vi "Set UI.vi"(6 "Lock":bool, 8 "error in (no error)":errorcluster, 10 "Available Tests":T6, 11 "Cluster":T1={"Queue Array"=[], "Queue Element"={"state"="", "data"=variant}, "System Event"=refnum, "System Event RefNum"=refnum, "Queue List"=[], "LPCA COM"="", "Rotating"=FALSE, "PrecorAI"="", "T_0 Index"=0, "Bar Graph X"=[], "Channels"=[], "Active Indicies"=[], "Active Channels"=[], "Sample Frequency"=0.0, "Ibrake Sweep"=[], "RPM Sweep"=[], "Load Sweep"=[], "Step Height Sweep"=[], "Range Sweep"=[], "A Counter"=0, "B Counter"=0, "C Counter"=0, "#A"=0, "#B"=0, "#C"=0, "Current RPM"=0.0, "Current Ibrake"=0, "Current Range"=0, "Current Step Height"=0, "Load Bank"=enum."OFF", "Cfg Cntrls"=[], "T_Monitor Indices"=[], "Thermal Limit"=0, "Thermal Resume"=0, "Timer Reset"=FALSE, "Stop Time"=0.0, "Autotest"=FALSE, "Pulsed RPM Capture"=FALSE, "Get Sample"=FALSE, "Last State"="", "Reset Timeout"=FALSE, "Ctrl Refs"={"Test Details"=refnum, "Save Config"=refnum, "Load Config"=refnum, "Path"=refnum, "Snapshot"=refnum, "SS#"=refnum, "Ibrake"=refnum, "RPM Target"=refnum, "Spin"=refnum, "Load Bank"=refnum, "Start Test"=refnum, "Pause Test"=refnum, "Load Sweep"=refnum, "RPM Sweep"=refnum, "Ibrake Sweep"=refnum, "Filters"=refnum, "Sample Frequency"=refnum, "Data Setup"=refnum, "Pause"=refnum, "Stop Time"=refnum, "S Period"=refnum, "Range"=refnum, "Step Height"=refnum, "Step Height Sweep"=refnum, "Range Sweep"=refnum, "Available Tests"=refnum, "RPM Graph"=refnum, "RPM Knob"=refnum, "FanMode"=refnum, "Fan Mode LED Array"=refnum, "Thermal Equilibrium"=refnum, "Data Display"=refnum, "LPCA Error"=refnum, "LPCA Ramp"=refnum, "LPCA Range"=refnum, "LPCA Resistance"=refnum, "Analyze Read"=refnum, "Console Select"=refnum, "Sub Panel"=refnum}, "Pulse Waveform"={"t0"=timestamp(0 s since 1904-01-01), "dt"=1.0, "Y"=[]}, "Snapshot"={"Test Details"="test", "Version"="test", "Date"=timestamp(3493915594.3018084 s since 1904-01-01), "Selected Test"="man", "Snapshot Number"=0, "Time"=timestamp(3493915602.7292905 s since 1904-01-01), "Ibrake Setpoint"="1", "RPM Setpoint"="20", "Range Setpoint"="", "Step Height Setpoint"="", "Load Bank Setpoint"="15", "Measurement Headers"="a,b,c,1,2,3", "Measurements"="1,2,3,4,5,6,7,8", "A"=0, "B"=0, "C"=0, "Raw Data"=[], "Available Tests"=enum."Manual", "Ibrake List"="", "RPM List"="", "Load Bank List"="", "Range List"="", "Step Height List"="", "FanMode Setpoint"=enum."Auto"}, "Sample Period"=0.0, "OverTemp"=FALSE, "Available Tests"=enum."Manual", "FanMode"=enum."Auto", "Fan Mode LED Array"=[FALSE, TRUE, FALSE], "Thermal\nEquilibrium "=FALSE, "Equilibrium Stop"=FALSE, "AvgDegChg"=[]} {"Snapshot"."Time" format="%<%H:%M:%S>T"; "Snapshot"."Date" format="%<%m/%d/%Y>T"}) -> (0 "error out":errorcluster)   [LabVIEW 2017]
uses:
  Controls/Available Tests.ctl
  Controls/Test TypeDef.ctl
  Code Library/Queue References Array.ctl
  Code Library/Queue Element.ctl
  Controls/Load Bank.ctl
  Console Sim/Controls/Console Select.ctl
  Controls/Snapshot Typedef.ctl
  Controls/FanMode.ctl
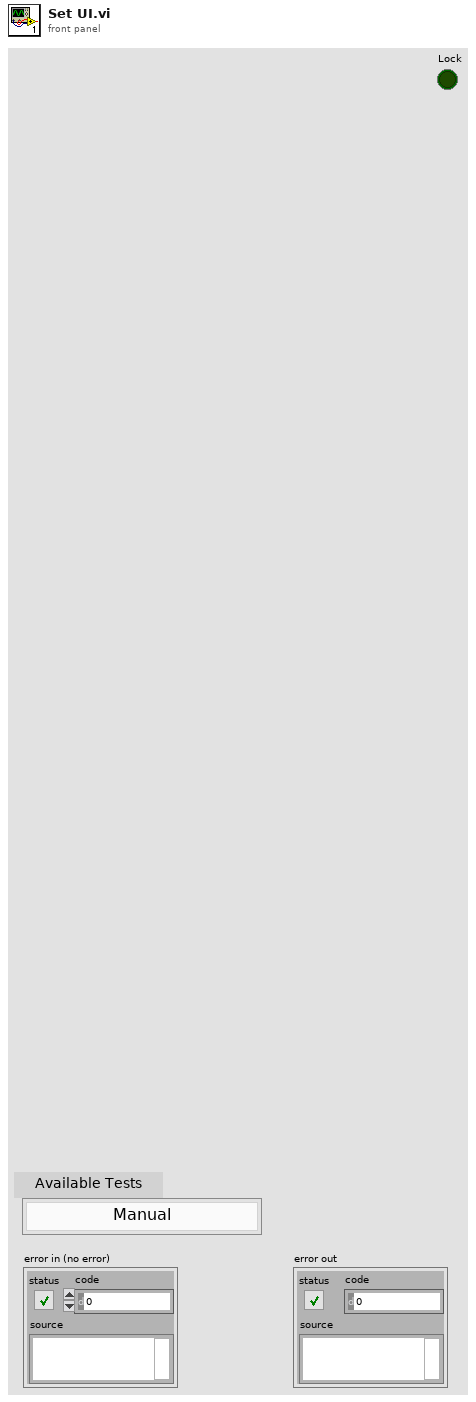
[diagram p1: front panel]
types:
  T1 = typedef "Test TypeDef.ctl" = cluster{"Queue Array":T2, "Queue Element":T3, "System Event":refnum<user-event>, "System Event RefNum":refnum<event-registration>, "Queue List":string[], "LPCA COM":refnum<visa-resource-name>, "Rotating":bool, "PrecorAI":refnum<k21>, "T_0 Index":i32, "Bar Graph X":i32[], "Channels":string[], "Active Indicies":i32[], "Active Channels":string[][], "Sample Frequency":dbl, "Ibrake Sweep":string[], "RPM Sweep":string[], "Load Sweep":string[], "Step Height Sweep":string[], "Range Sweep":string[], "A Counter":i32, "B Counter":i32, "C Counter":i32, "#A":i32, "#B":i32, "#C":i32, "Current RPM":dbl, "Current Ibrake":u32, "Current Range":u32, "Current Step Height":u32, "Load Bank":T4, "Cfg Cntrls":refnum<vi>[], "T_Monitor Indices":i32[], "Thermal Limit":i32, "Thermal Resume":i32, "Timer Reset":bool, "Stop Time":dbl, "Autotest":bool, "Pulsed RPM Capture":bool, "Get Sample":bool, "Last State":string, "Reset Timeout":bool, "Ctrl Refs":cluster{"Test Details":refnum<vi>, "Save Config":refnum<vi>, "Load Config":refnum<vi>, "Path":refnum<vi>, "Snapshot":refnum<vi>, "SS#":refnum<vi>, "Ibrake":refnum<vi>, "RPM Target":refnum<vi>, "Spin":refnum<vi>, "Load Bank":refnum<vi>, "Start Test":refnum<vi>, "Pause Test":refnum<vi>, "Load Sweep":refnum<vi>, "RPM Sweep":refnum<vi>, "Ibrake Sweep":refnum<vi>, "Filters":refnum<vi>, "Sample Frequency":refnum<vi>, "Data Setup":refnum<vi>, "Pause":refnum<vi>, "Stop Time":refnum<vi>, "S Period":refnum<vi>, "Range":refnum<vi>, "Step Height":refnum<vi>, "Step Height Sweep":refnum<vi>, "Range Sweep":refnum<vi>, "Available Tests":refnum<vi>, "RPM Graph":refnum<vi>, "RPM Knob":refnum<vi>, "FanMode":refnum<vi>, "Fan Mode LED Array":refnum<vi>, "Thermal Equilibrium":refnum<vi>, "Data Display":refnum<vi>, "LPCA Error":refnum<vi>, "LPCA Ramp":refnum<vi>, "LPCA Range":refnum<vi>, "LPCA Resistance":refnum<vi>, "Analyze Read":refnum<vi>, "Console Select":refnum<vi>, "Sub Panel":refnum<vi>}, "Pulse Waveform":waveform(dbl), "Snapshot":T5, "Sample Period":dbl, "OverTemp":bool, "Available Tests":T6, "FanMode":T7, "Fan Mode LED Array":bool[], "Thermal\nEquilibrium ":bool, "Equilibrium Stop":bool, "AvgDegChg":dbl[]}
  T2 = typedef "Queue References Array.ctl" = refnum<queue>[]
  T3 = typedef "Queue Element.ctl" = cluster{"state":string, "data":variant}
  T4 = typedef "Load Bank.ctl" = enum16{"OFF", "50", "25", "16.7", "12.5", "10.0", "8.3", "7.1", "6.3", "5.6", "5.0", "4.5", "4.2", "3.8", "3.6", "3.3", "3.1"}
  T5 = typedef "Snapshot Typedef.ctl" = cluster{"Test Details":string, "Version":string, "Date":timestamp, "Selected Test":string, "Snapshot Number":u16, "Time":timestamp, "Ibrake Setpoint":string, "RPM Setpoint":string, "Range Setpoint":string, "Step Height Setpoint":string, "Load Bank Setpoint":string, "Measurement Headers":string, "Measurements":string, "A":i32, "B":i32, "C":i32, "Raw Data":string[][], "Available Tests":T6, "Ibrake List":string, "RPM List":string, "Load Bank List":string, "Range List":string, "Step Height List":string, "FanMode Setpoint":T7}
  T6 = typedef "Available Tests.ctl" = enum16{"Manual", "EFX Brake Torque", "Generator Torque", "EFX Brake Thermal", "Generator Thermal", "Pulsed RPM", "AMT Brake Torque", "Bike Brake Torque", "AMT Brake Thermal", "Bike Brake Thermal"}
  T7 = typedef "FanMode.ctl" = enum16{"On", "Off", "Auto"}
  T8 = enum8{"Enabled", "Disabled", "Disabled and Grayed Out"}
  T9 = cluster{"Test Details":refnum<vi>, "Save Config":refnum<vi>, "Load Config":refnum<vi>, "Path":refnum<vi>, "Snapshot":refnum<vi>, "SS#":refnum<vi>, "Ibrake":refnum<vi>, "RPM Target":refnum<vi>, "Spin":refnum<vi>, "Load Bank":refnum<vi>, "Start Test":refnum<vi>, "Pause Test":refnum<vi>, "Load Sweep":refnum<vi>, "RPM Sweep":refnum<vi>, "Ibrake Sweep":refnum<vi>, "Filters":refnum<vi>, "Sample Frequency":refnum<vi>, "Data Setup":refnum<vi>, "Pause":refnum<vi>, "Stop Time":refnum<vi>, "S Period":refnum<vi>, "Range":refnum<vi>, "Step Height":refnum<vi>, "Step Height Sweep":refnum<vi>, "Range Sweep":refnum<vi>, "Available Tests":refnum<vi>, "RPM Graph":refnum<vi>, "RPM Knob":refnum<vi>, "FanMode":refnum<vi>, "Fan Mode LED Array":refnum<vi>, "Thermal Equilibrium":refnum<vi>, "Data Display":refnum<vi>, "LPCA Error":refnum<vi>, "LPCA Ramp":refnum<vi>, "LPCA Range":refnum<vi>, "LPCA Resistance":refnum<vi>, "Analyze Read":refnum<vi>, "Console Select":refnum<vi>, "Sub Panel":refnum<vi>}
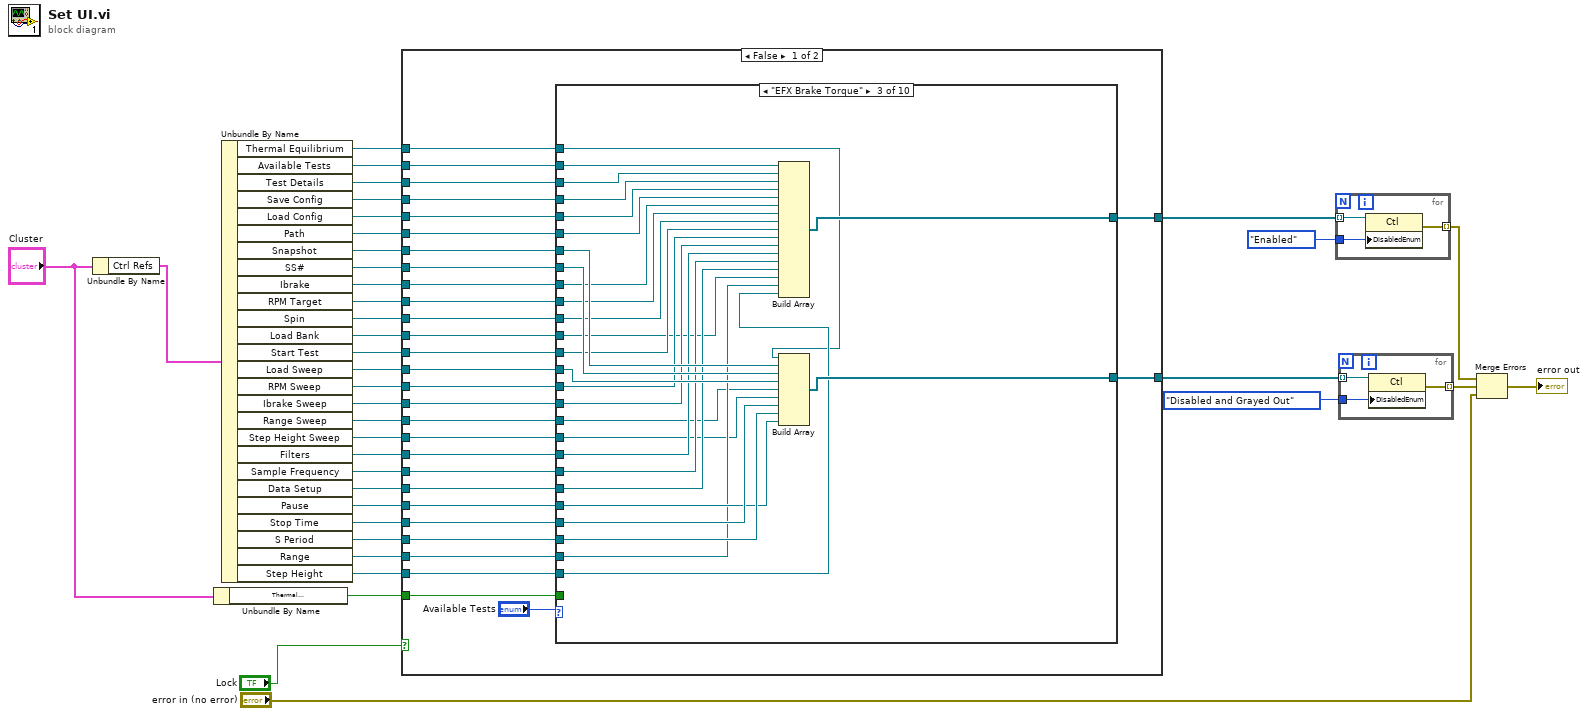
[diagram p0: block diagram]
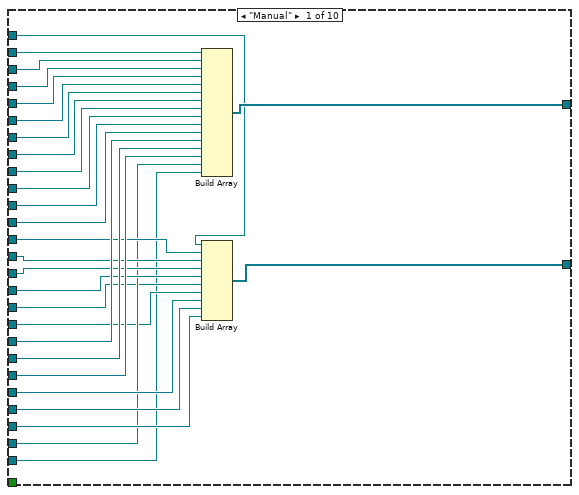
[diagram p2: hidden frame]
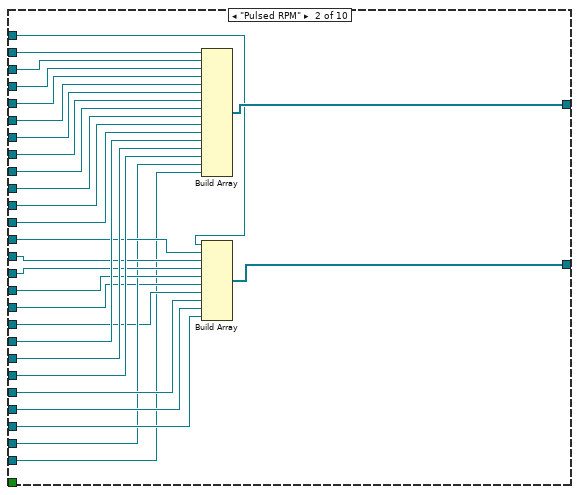
[diagram p3: hidden frame]
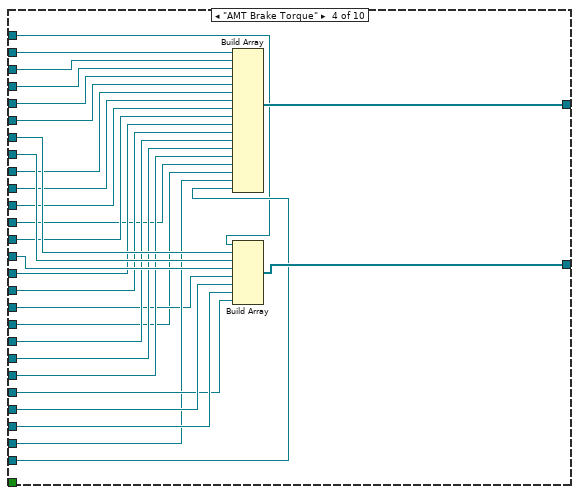
[diagram p4: hidden frame]
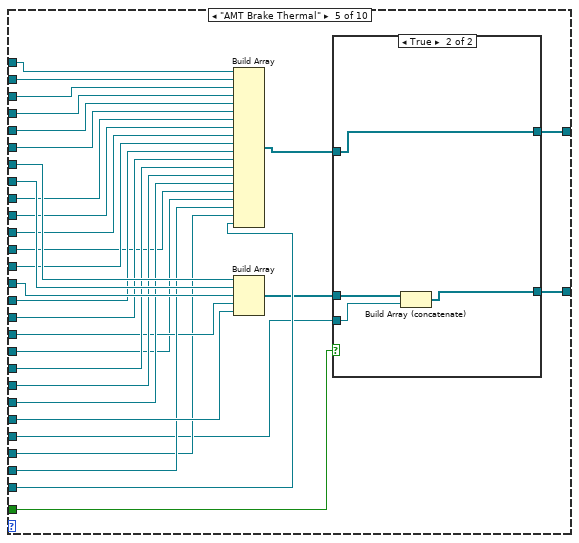
[diagram p5: hidden frame]
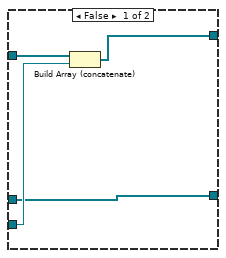
[diagram p6: hidden frame]
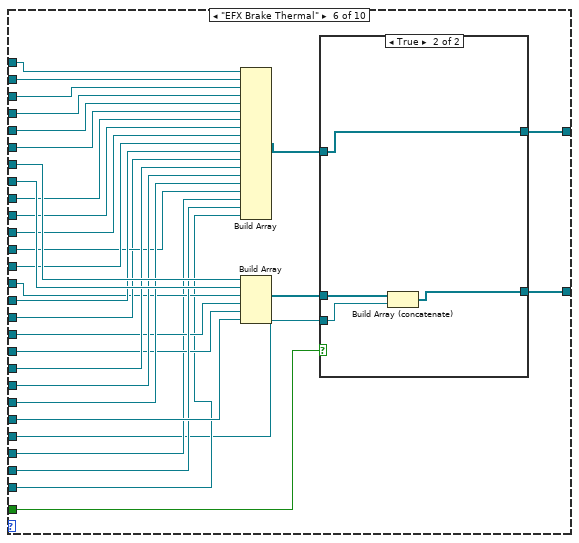
[diagram p7: hidden frame]
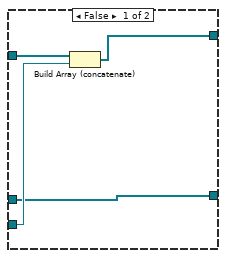
[diagram p8: hidden frame]
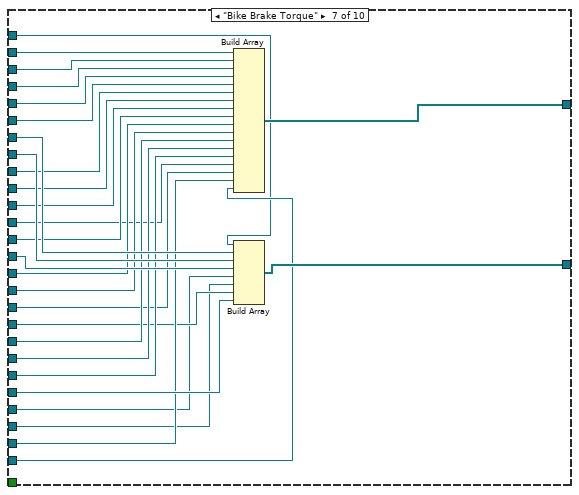
[diagram p9: hidden frame]
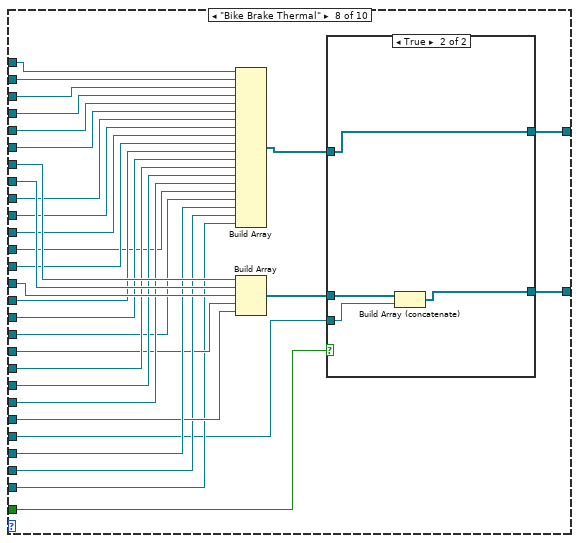
[diagram p10: hidden frame]
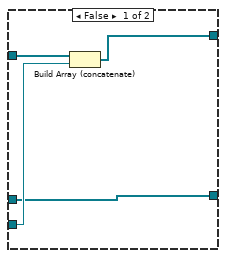
[diagram p11: hidden frame]
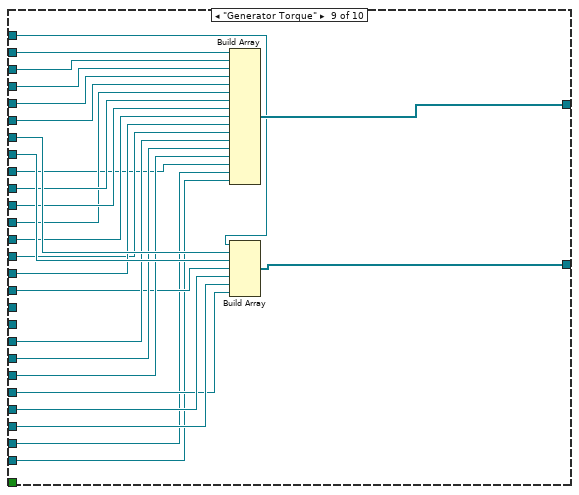
[diagram p12: hidden frame]
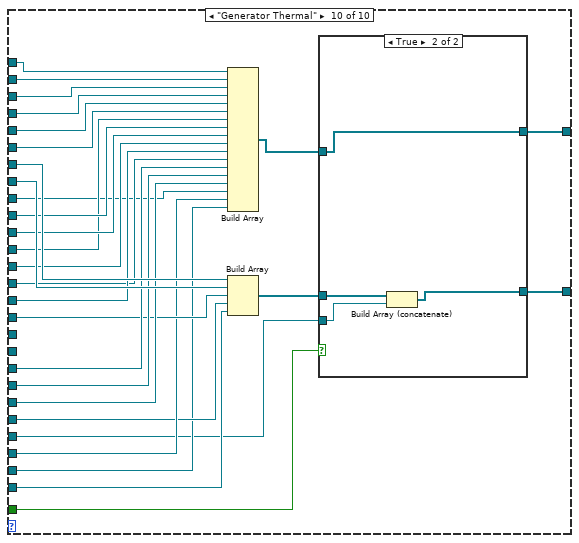
[diagram p13: hidden frame]
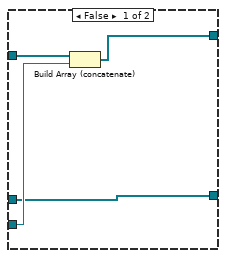
[diagram p14: hidden frame]
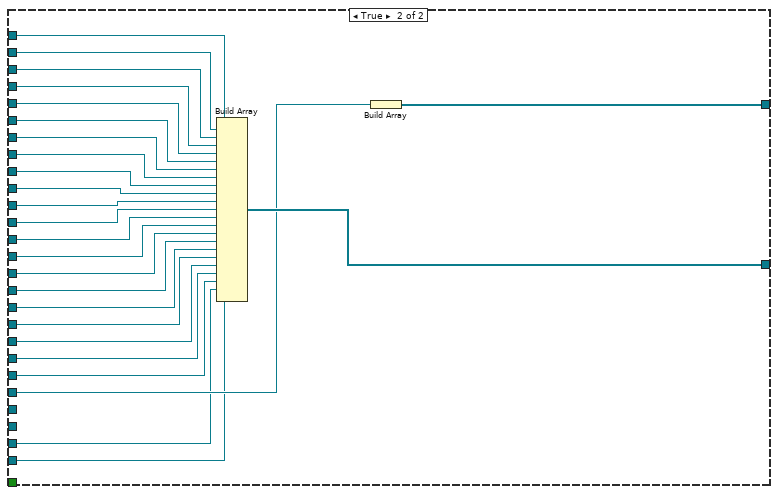
[diagram p15: hidden frame]
diagram:
  n1 = Unbundle By Name("Cluster") -> ("Ctrl Refs"=w7:T9)
  n2 = Unbundle By Name("Cluster") -> ("Thermal\nEquilibrium"=w4:bool)
  n3 = Unbundle By Name(w7) -> ("Thermal Equilibrium"=w1:refnum<vi>, "Available Tests"=w22:refnum<vi>, "Test Details"=w23:refnum<vi>, "Save Config"=w24:refnum<vi>, "Load Config"=w25:refnum<vi>, "Path"=w26:refnum<vi>, "Snapshot"=w27:refnum<vi>, "SS#"=w28:refnum<vi>, "Ibrake"=w29:refnum<vi>, "RPM Target"=w30:refnum<vi>, "Spin"=w31:refnum<vi>, "Load Bank"=w32:refnum<vi>, "Start Test"=w33:refnum<vi>, "Load Sweep"=w34:refnum<vi>, "RPM Sweep"=w35:refnum<vi>, "Ibrake Sweep"=w36:refnum<vi>, "Range Sweep"=w10:refnum<vi>, "Step Height Sweep"=w9:refnum<vi>, "Filters"=w11:refnum<vi>, "Sample Frequency"=w37:refnum<vi>, "Data Setup"=w38:refnum<vi>, "Pause"=w15:refnum<vi>, "Stop Time"=w14:refnum<vi>, "S Period"=w13:refnum<vi>, "Range"=w12:refnum<vi>, "Step Height"=w8:refnum<vi>)
  n4 = case shown="False" "Lock" {
    tunnel: w38 -> [w68 w413]
    tunnel: w37 -> [w67 w411]
    tunnel: w11 -> [w66 w409]
    tunnel: w36 -> [w65 w407]
    tunnel: w35 -> [w64 w405]
    tunnel: w34 -> [w63 w403]
    tunnel: w33 -> [w62 w401]
    tunnel: w32 -> [w61 w400]
    tunnel: w31 -> [w60 w397]
    tunnel: w30 -> [w59 w398]
    tunnel: w29 -> [w58 w399]
    tunnel: w28 -> [w57 w402]
    tunnel: w27 -> [w56 w404]
    tunnel: w26 -> [w55 w406]
    tunnel: w25 -> [w54 w408]
    tunnel: w24 -> [w53 w410]
    tunnel: w23 -> [w52 w412]
    tunnel: w22 -> [w51 w414]
    tunnel: [w50 w396] -> w19
    tunnel: [w49 w394] -> w3
    tunnel: w15 -> [w48 w395]
    tunnel: w14 -> [w47 _]
    tunnel: w13 -> [w46 _]
    tunnel: w12 -> [w45 w393]
    tunnel: w10 -> [w44 w392]
    tunnel: w9 -> [w43 w391]
    tunnel: w8 -> [w42 w390]
    tunnel: w4 -> [w40 _]
    tunnel: w1 -> [w39 w389]
    frame False {
      n5 = case shown="\"EFX Brake Torque\"" "Available Tests" {
        tunnel: w51 -> [w96 w124 w148 w176 w208 w248 w282 w314 w348 w378]
        tunnel: w52 -> [w95 w123 w147 w175 w207 w247 w281 w313 w347 w377]
        tunnel: w53 -> [w94 w122 w146 w174 w206 w246 w280 w312 w346 w376]
        tunnel: w54 -> [w93 w121 w145 w173 w205 w245 w279 w311 w345 w375]
        tunnel: w55 -> [w92 w120 w144 w172 w204 w244 w278 w310 w344 w374]
        tunnel: w56 -> [w91 w119 w152 w180 w211 w250 w286 w317 w351 w380]
        tunnel: w57 -> [w90 w118 w151 w179 w210 w249 w285 w316 w350 w379]
        tunnel: w58 -> [w89 w117 w143 w171 w203 w243 w277 w309 w332 w363]
        tunnel: w59 -> [w88 w116 w142 w170 w202 w242 w276 w308 w343 w373]
        tunnel: w60 -> [w87 w115 w141 w169 w201 w241 w275 w307 w342 w372]
        tunnel: w61 -> [w86 w114 w133 w161 w194 w235 w267 w300 w334 w365]
        tunnel: w62 -> [w82 w110 w140 w168 w200 w240 w274 w306 w341 w371]
        tunnel: w63 -> [w81 w109 w150 w178 w209 w229 w284 w315 w333 w364]
        tunnel: w64 -> [w80 w108 w139 w167 w199 w239 w273 w305 w340 w370]
        tunnel: w65 -> [w79 w107 w138 w166 w198 w230 w272 w304 w335 w366]
        tunnel: w66 -> [w85 w113 w137 w165 w197 w238 w271 w303 w339 w369]
        tunnel: w67 -> [w84 w112 w136 w164 w196 w237 w270 w302 w338 w368]
        tunnel: w68 -> [w83 w111 w135 w163 w195 w236 w269 w301 w337 w367]
        tunnel: [w78 w106 w149 w177 w182 w221 w283 w288 w349 w358] -> w50
        tunnel: [w77 w105 w134 w162 w183 w222 w268 w289 w336 w357] -> w49
        tunnel: w48 -> [w76 w104 w130 w158 w193 w234 w266 w298 w329 w361]
        tunnel: w47 -> [w75 w103 w132 w160 w184 w224 w261 w292 w331 w355]
        tunnel: w46 -> [w74 w102 w131 w159 w189 w228 w262 w299 w330 w362]
        tunnel: w45 -> [w73 w101 w129 w157 w192 w233 w265 w297 w328 w360]
        tunnel: w44 -> [w72 w100 w127 w156 w191 w232 w263 w295 _ _]
        tunnel: w43 -> [w71 w99 w128 w155 w190 w231 w264 w296 _ _]
        tunnel: w42 -> [w70 w98 w126 w154 w188 w227 w260 w294 w327 w359]
        tunnel: w40 -> [_ _ _ _ w187 w223 _ w293 _ w356]
        tunnel: w39 -> [w69 w97 w125 w153 w181 w220 w259 w287 w326 w352]
        frame "Manual" {
          n6 = Build Array(w96, w95, w94, w93, w92, w91, w90, w89, w88, w87, w86, w85, w84, w83, w73, w70) -> (w77:refnum<vi>[])
          n7 = Build Array(w69, w82, w81, w80, w79, w72, w71, w76, w75, w74) -> (w78:refnum<vi>[])
        }
        frame "Pulsed RPM" {
          n8 = Build Array(w124, w123, w122, w121, w120, w119, w118, w117, w116, w115, w114, w113, w112, w111, w101, w98) -> (w105:refnum<vi>[])
          n9 = Build Array(w97, w110, w109, w108, w107, w100, w99, w104, w103, w102) -> (w106:refnum<vi>[])
        }
        frame "EFX Brake Torque" {
          n10 = Build Array(w148, w147, w146, w145, w144, w143, w142, w141, w140, w139, w138, w137, w136, w135, w133, w129, w126) -> (w134:refnum<vi>[])
          n11 = Build Array(w125, w152, w151, w150, w127, w128, w132, w131, w130) -> (w149:refnum<vi>[])
        }
        frame "AMT Brake Torque" {
          n12 = Build Array(w176, w175, w174, w173, w172, w171, w170, w169, w168, w167, w166, w165, w164, w163, w161, w155, w157, w154) -> (w162:refnum<vi>[])
          n13 = Build Array(w153, w180, w179, w178, w156, w160, w159, w158) -> (w177:refnum<vi>[])
        }
        frame "AMT Brake Thermal" {
          n14 = Build Array(w181, w208, w207, w206, w205, w204, w203, w202, w201, w200, w199, w198, w197, w196, w195, w194, w190, w192, w189, w188) -> (w186:refnum<vi>[])
          n15 = Build Array(w211, w210, w209, w191, w193) -> (w185:refnum<vi>[])
          n16 = case shown="True" w187 {
            tunnel: w186 -> [w215 w217]
            tunnel: w185 -> [w212 w219]
            tunnel: w184 -> [w214 w218]
            tunnel: [w213 w217] -> w183
            tunnel: [w212 w216] -> w182
            frame False {
              n17 = Build Array (concatenate)(w215, w214) -> (w213:refnum<vi>[])
            }
            frame True {
              n18 = Build Array (concatenate)(w219, w218) -> (w216:refnum<vi>[])
            }
          }
        }
        frame "EFX Brake Thermal" {
          n19 = Build Array(w220, w248, w247, w246, w245, w244, w243, w242, w241, w240, w239, w230, w238, w237, w236, w235, w228, w233, w227) -> (w226:refnum<vi>[])
          n20 = Build Array(w250, w249, w229, w232, w231, w234) -> (w225:refnum<vi>[])
          n21 = case shown="True" w223 {
            tunnel: w226 -> [w254 w256]
            tunnel: w225 -> [w251 w258]
            tunnel: w224 -> [w253 w257]
            tunnel: [w252 w256] -> w222
            tunnel: [w251 w255] -> w221
            frame False {
              n22 = Build Array (concatenate)(w254, w253) -> (w252:refnum<vi>[])
            }
            frame True {
              n23 = Build Array (concatenate)(w258, w257) -> (w255:refnum<vi>[])
            }
          }
        }
        frame "Bike Brake Torque" {
          n24 = Build Array(w282, w281, w280, w279, w278, w277, w276, w275, w274, w273, w272, w271, w270, w269, w267, w263, w265, w260) -> (w268:refnum<vi>[])
          n25 = Build Array(w259, w286, w285, w284, w261, w262, w264, w266) -> (w283:refnum<vi>[])
        }
        frame "Bike Brake Thermal" {
          n26 = Build Array(w287, w314, w313, w312, w311, w310, w309, w308, w307, w306, w305, w304, w303, w302, w301, w300, w295, w299, w297, w294) -> (w290:refnum<vi>[])
          n27 = Build Array(w317, w316, w315, w296, w298) -> (w291:refnum<vi>[])
          n28 = case shown="True" w293 {
            tunnel: w290 -> [w321 w323]
            tunnel: w291 -> [w318 w325]
            tunnel: w292 -> [w320 w324]
            tunnel: [w319 w323] -> w289
            tunnel: [w318 w322] -> w288
            frame False {
              n29 = Build Array (concatenate)(w321, w320) -> (w319:refnum<vi>[])
            }
            frame True {
              n30 = Build Array (concatenate)(w325, w324) -> (w322:refnum<vi>[])
            }
          }
        }
        frame "Generator Torque" {
          n31 = Build Array(w348, w347, w346, w345, w344, w334, w343, w342, w341, w340, w333, w339, w338, w337, w332, w328, w327) -> (w336:refnum<vi>[])
          n32 = Build Array(w326, w351, w350, w335, w331, w330, w329) -> (w349:refnum<vi>[])
        }
        frame "Generator Thermal" {
          n33 = Build Array(w352, w378, w377, w376, w375, w374, w365, w373, w372, w371, w370, w364, w369, w368, w367, w363, w362, w360) -> (w353:refnum<vi>[])
          n34 = Build Array(w380, w379, w366, w361, w359) -> (w354:refnum<vi>[])
          n35 = case shown="True" w356 {
            tunnel: w353 -> [w384 w386]
            tunnel: w354 -> [w381 w388]
            tunnel: w355 -> [w383 w387]
            tunnel: [w382 w386] -> w357
            tunnel: [w381 w385] -> w358
            frame False {
              n36 = Build Array (concatenate)(w384, w383) -> (w382:refnum<vi>[])
            }
            frame True {
              n37 = Build Array (concatenate)(w388, w387) -> (w385:refnum<vi>[])
            }
          }
        }
      }
    }
    frame True {
      n38 = Build Array(w389, w414, w412, w410, w408, w406, w404, w402, w399, w398, w397, w400, w401, w403, w405, w407, w392, w391, w409, w411, w413, w393, w390) -> (w396:refnum<vi>[])
      n39 = Build Array(w395) -> (w394:refnum<vi>[])
    }
  }
  n40 = for {
    tunnel: [w417] -> w2 mode=indexing
    tunnel: w3 -> [w416] mode=indexing
    tunnel: T8."Enabled" ("Disabled") -> [w415]
    n41 = property class="Ctl"(reference=w416, "DisabledEnum"=w415) -> (error out=w417:errorcluster)  [unwired: 1 in, 1 out]
  }
  n42 = for {
    tunnel: [w420] -> w20 mode=indexing
    tunnel: w19 -> [w419] mode=indexing
    tunnel: T8."Disabled and Grayed Out" ("Disabled") -> [w418]
    n43 = property class="Ctl"(reference=w419, "DisabledEnum"=w418) -> (error out=w420:errorcluster)  [unwired: 1 in, 1 out]
  }
  n44 = Merge Errors(w2, w20, "error in (no error)") -> (→"error out":errorcluster)
